vi "String - XML String Encoding.vi"(11 "HEX String":string) -> (3 "XML String":string)   [LabVIEW 2013]
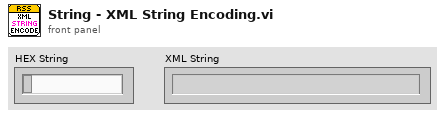
[diagram p1: front panel]
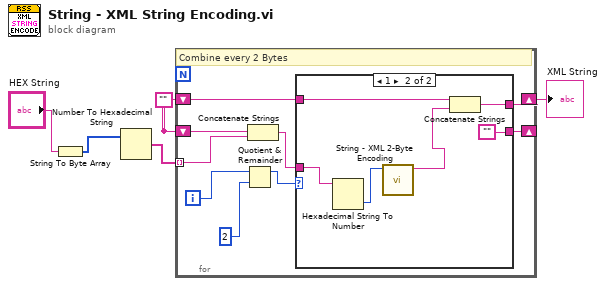
[diagram p0: block diagram]
diagram:
  w4 = ""
  n1 = String To Byte Array(string="HEX String") -> (unsigned byte array=w1:u8[])
  n2 = Number To Hexadecimal String(2:w1) -> (0:w2:string[])  [unwired: 1 in]
  n3 = for {
    shift-right: [w8] -> _
    shift-left: w4 -> [w13]
    tunnel: w2 -> [w14] mode=indexing
    shift-right: [w6] -> w5
    shift-left: w4 -> [w7]
    i -> [w12]
    # "Combine every 2 Bytes"
    n4 = Quotient & Remainder(x=w12, y=2) -> (x-y*floor(x/y)=w10:i32)  [unwired: 1 out]
    n5 = Concatenate Strings(w13, w14) -> (w9:string)
    n6 = case shown="1" w10 {
      tunnel: w9 -> [w16 w18]
      tunnel: [w16 ""] -> w8
      tunnel: w7 -> [w15 w21]
      tunnel: [w15 w19] -> w6
      frame 0, Default {
      }
      frame 1 {
        n7 = Hexadecimal String To Number(string=w18) -> (number=w17:u32)  [unwired: 2 in, 1 out]
        n8 = call "String - XML 2-Byte Encoding.vi"("Number In (2-Bytes -16bits)"=w17) -> ("Output (/ Format)"=w20:string)  [unwired: 7 in, 2 out]
        n9 = Concatenate Strings(w21, w20) -> (w19:string)
      }
    }
  }
  "XML String" <- w5
